vi "Run RT Sequence.vi"(0 "Sequence Context":T1, 1 "RT Sequence File Path":path, 2 "Gateway IP Address":string, 3 "Target (\"\": Auto-assign)":string, 4 "Sequence Timeout (s)":i32=10000, 5 "Step Timeout (ms)":dbl=10000.0, 6 "ParamNames":string[](array[string]), 7 "NumericDataType":string, 8 "ParamValues":string[](array[string]), 10 "ParamTypes":string[](array[string])) -> (14 "Report Text":string, 15 "Numeric Return Value":dbl, 16 "PassFail Return Value":bool, 17 "RT Sequence File Path out":path, 19 "error out":errorcluster)   [LabVIEW 2020, in "ni-veristand-steps-runtime-lib.lvlib"]
uses:
  ni-veristand-steps-runtime-lib.lvlib
  <vilib>/addons/TestStand/_TSLegacy.llb/LabVIEW Test - Sequence Context.ctl
  NationalInstruments.VeriStand.DataTypes
  <vilib>/NI VeriStand/Execution/SequenceExecutionInterface/Sequence Execution State.ctl
  <vilib>/NI VeriStand/Execution/SequenceExecutionInterface/NI_VS Sequence Execution Interface.lvlib
panel:
  out "Session Name out":string
  out "ms time elapsed (debug)":u32
  out "Timed out?":bool
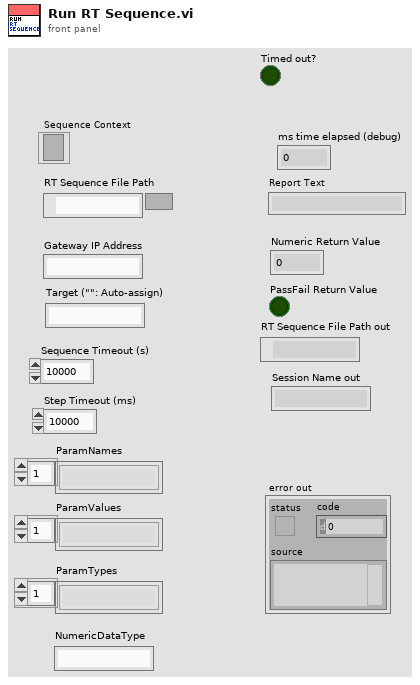
[diagram p1: front panel]
types:
  T1 = typedef "LabVIEW Test - Sequence Context.ctl" = refnum<k7>
  T2 = typedef "NI_VS Sequence Execution Interface.lvlib/Sequence Input Assignment Ref.ctl" = refnum<k24>
  T3 = typedef "NI_VS Sequence Execution Interface.lvlib/Sequence Call Ref.ctl" = refnum<k24>
  T4 = typedef "NI_VS Sequence Execution Interface.lvlib/Stimulus Profile Session Ref.ctl" = refnum<k24>
  T5 = typedef "TestStand - Status Monitor.ctl" = cluster{"Sequence Context":refnum<k7>, "Execution":refnum<k7>, "Termination Monitor":refnum<k7>}
  T6 = typedef "NI_VS Sequence Execution Interface.lvlib/Sequence Execution State.ctl" = enum16{"Idle", "Running", "SingleStepping", "Paused", "Stopped"}
  T7 = typedef "NI_VS Sequence Execution Interface.lvlib/Data Value Ref.ctl" = refnum<k24>
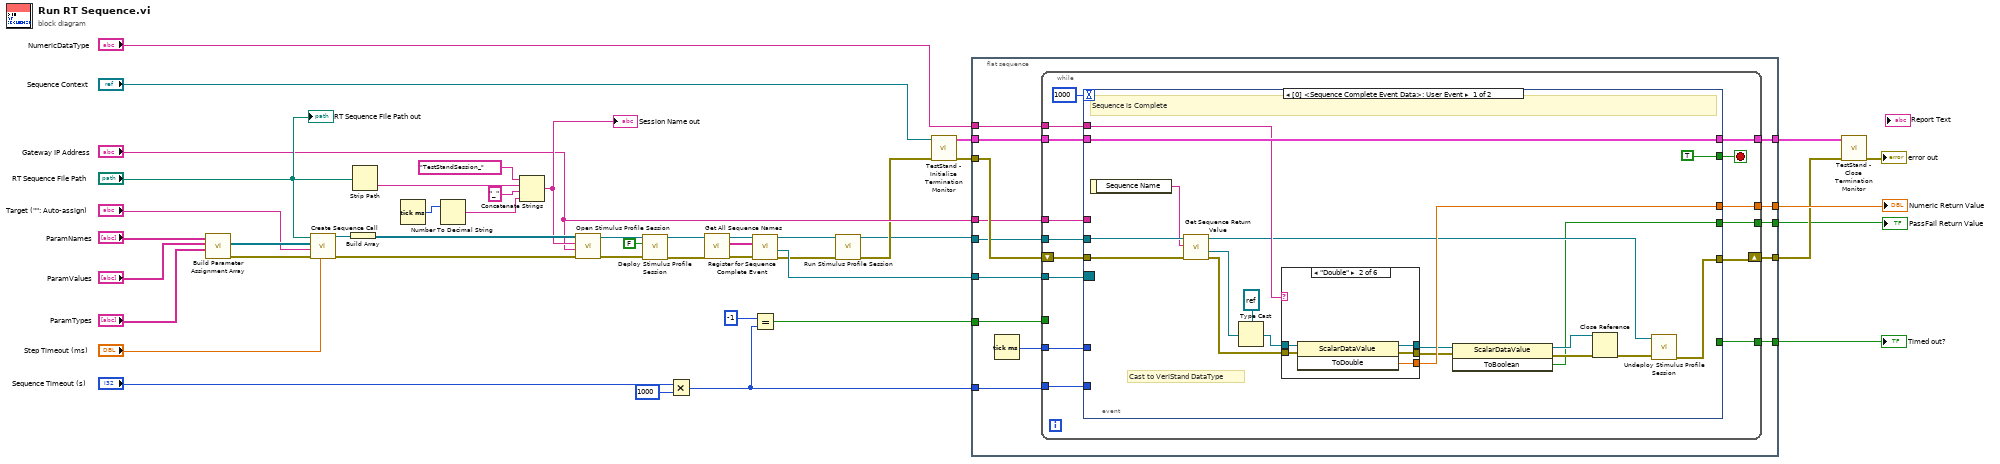
[diagram p0: block diagram]
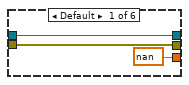
[diagram p2: hidden frame]
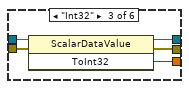
[diagram p3: hidden frame]
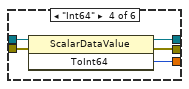
[diagram p4: hidden frame]
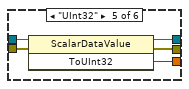
[diagram p5: hidden frame]
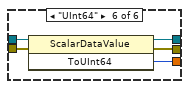
[diagram p6: hidden frame]
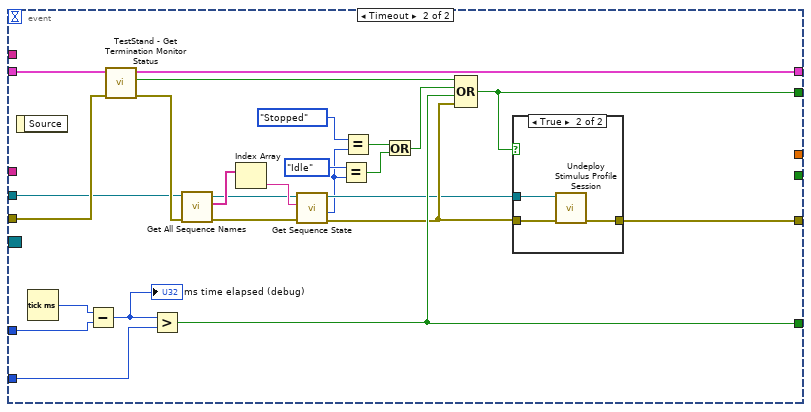
[diagram p7: hidden frame]
diagram:
  n1 = call "Build Parameter Assignment Array.vi"("ParamTypes"="ParamTypes", "ParamValues"="ParamValues", "ParamNames"="ParamNames") -> ("error out"=w43:errorcluster, "Sequence Parameter Assignment refs"=w42:T2[])  [unwired: 7 in]
  n2 = call <vilib>:"Create Sequence Call.vi"("Timeout ms (10000)"="Step Timeout (ms)", "error in (no error)"=w43, "Target (\"\": Auto-assign)"="Target (\"\": Auto-assign)", "Parameter Assignments"=w42, "Sequence File Path"="RT Sequence File Path") -> ("error out"=w11:errorcluster, "Sequence Call Ref"=w40:T3)  [unwired: 5 in]
  n3 = Build Array(w40) -> (w39:T3[])
  n4 = Strip Path(path="RT Sequence File Path") -> (name=w12:string)  [unwired: 1 out]
  n5 = Tick Count (ms)() -> (millisecond timer value=w8:u32)
  n6 = Number To Decimal String(number=w8) -> (decimal integer string=w7:string)  [unwired: 1 in]
  n7 = Concatenate Strings("TestStandSession_" ("Session Name"), w12, "_" ("string"), w7) -> (w14:string)
  "Session Name out" <- w14
  n8 = call <vilib>:"Open Stimulus Profile Session.vi"("error in (no error)"=w11, "Gateway IP Address (\"\": localhost)"="Gateway IP Address", "Session Name"=w14, "Sequence Calls"=w39) -> ("error out"=w36:errorcluster, "Session Ref"=w37:T4)  [unwired: 6 in]
  n9 = call <vilib>:"Deploy Stimulus Profile Session.vi"("error in (no error)"=w36, "Auto-Start (T)"=FALSE, "Session Ref in"=w37) -> ("error out"=w35:errorcluster, "Session Ref out"=w34:T4)  [unwired: 6 in, 1 out]
  n10 = Multiply(x="Sequence Timeout (s)", y=1000) -> (x*y=w26:i32)
  n11 = call <vilib>:"Get All Sequence Names.vi"("error in (no error)"=w35, "Session Ref in"=w34) -> ("error out"=w24:errorcluster, "Sequence Names out"=w22:string[], "Session Ref out"=w23:T4)  [unwired: 7 in]
  n12 = call <vilib>:"Register for Sequence Complete Event.vi"("error in (no error)"=w24, "Sequence Names"=w22, "Session Ref in"=w23) -> ("error out"=w3:errorcluster, "Event Registration Refnum"=w9:refnum<event-registration>, "Session Ref out"=w4:T4)  [unwired: 4 in, 2 out]
  n13 = Equal?(x=-1, y=w26) -> (x = y?=w29:bool)
  n14 = call <vilib>:"Run Stimulus Profile Session.vi"("error in (no error)"=w3, "Session Ref in"=w4) -> ("error out"=w2:errorcluster, "Session Ref out"=w1:T4)  [unwired: 8 in]
  n15 = call <vilib>:"TestStand - Initialize Termination Monitor.vi"("error in (no error)"=w2, "Sequence Context In"="Sequence Context") -> ("error out"=w32:errorcluster, "Status Monitor Out"=w31:T5)  [unwired: 8 in]
  n16 = flat-sequence {
    tunnel: w32 -> [w60]
    tunnel: w31 -> [w59]
    tunnel: w29 -> [w58]
    tunnel: w26 -> [w57]
    tunnel: w1 -> [w56]
    tunnel: w9 -> [w55]
    tunnel: [w54] -> w18
    tunnel: [w53] -> w21
    tunnel: "NumericDataType" -> [w51]
    tunnel: [w50] -> w19
    tunnel: [w49] -> w16
    tunnel: [w48] -> w17
    tunnel: "Gateway IP Address" -> [w47]
    frame #0 {
      n17 = Tick Count (ms)() -> (millisecond timer value=w52:u32)
      n18 = while {
        tunnel: w59 -> [w69]
        tunnel: w57 -> [w66]
        tunnel: w58 -> [_]
        shift-right: [w71] -> w54
        shift-left: w60 -> [w75]
        tunnel: w56 -> [w74]
        tunnel: w55 -> [w73]
        tunnel: [w68] -> w53
        tunnel: w52 -> [w67]
        tunnel: w51 -> [w65]
        tunnel: [w64] -> w50
        tunnel: [w63] -> w49
        tunnel: [w62] -> w48
        tunnel: w47 -> [w61]
        stop <- w72 stop-if-true
        n19 = event shown="[0] <Sequence Complete Event Data>: User Event" {
          selector: w73 -> [_ _]
          dyn-events: _ -> [_ _]
          timeout: 1000 -> [_ _]
          tunnel: w75 -> [w92 w146]
          tunnel: w74 -> [w91 w135]
          tunnel: [TRUE w137] -> w72
          tunnel: [w77 w138] -> w71
          tunnel: w69 -> [w93 w147]
          tunnel: [w93 w145] -> w68
          tunnel: w67 -> [_ w143]
          tunnel: w66 -> [_ w141]
          tunnel: w65 -> [w85 _]
          tunnel: [w84 _] -> w64
          tunnel: [w76 _] -> w63
          tunnel: [_ w139] -> w62
          tunnel: w61 -> [_ _]
          event User Event {
            # "Cast to VeriStand DataType"
            # "Sequence is Complete"
            n20 = event-data() -> ("Sequence Name"=w90:string)  [unwired: 1 in]
            n21 = call <vilib>:"Get Sequence Return Value.vi"("error in (no error)"=w92, "Sequence Name"=w90, "Session Ref in"=w91) -> ("error out"=w87:errorcluster, "Data Value Ref"=w88:T7, "Session Ref out"=w78:T4)  [unwired: 5 in, 1 out]
            n22 = Type Cast(type=refnum<k24> refnum ("Node"), x=w88) -> (*(type *) &x=w86:refnum<k24>)
            n23 = case shown="\"Double\"" w85 {
              tunnel: [w95 w102 w107 w112 w117 w122] -> w83
              tunnel: [w96 w101 w106 w111 w116 w121] -> w82
              tunnel: [nan ("ToDouble") w100 w105 w110 w115 w118] -> w84
              tunnel: w86 -> [w96 w99 w103 w109 w113 w119]
              tunnel: w87 -> [w95 w98 w104 w108 w114 w120]
              frame Default {
              }
              frame "Double" {
                n24 = invoke class="ScalarDataValue" method="ToDouble"(reference=w99, error in=w98) -> (reference out=w101:refnum<k24>, error out=w102:errorcluster, "ToDouble"=w100:dbl)  [unwired: 1 in]
              }
              frame "Int32" {
                n25 = invoke class="ScalarDataValue" method="ToInt32"(reference=w103, error in=w104) -> (reference out=w106:refnum<k24>, error out=w107:errorcluster, "ToInt32"=w105:i32)  [unwired: 1 in]
              }
              frame "Int64" {
                n26 = invoke class="ScalarDataValue" method="ToInt64"(reference=w109, error in=w108) -> (reference out=w111:refnum<k24>, error out=w112:errorcluster, "ToInt64"=w110:i64)  [unwired: 1 in]
              }
              frame "UInt32" {
                n27 = invoke class="ScalarDataValue" method="ToUInt32"(reference=w113, error in=w114) -> (reference out=w116:refnum<k24>, error out=w117:errorcluster, "ToUInt32"=w115:u32)  [unwired: 1 in]
              }
              frame "UInt64" {
                n28 = invoke class="ScalarDataValue" method="ToUInt64"(reference=w119, error in=w120) -> (reference out=w121:refnum<k24>, error out=w122:errorcluster, "ToUInt64"=w118:u64)  [unwired: 1 in]
              }
            }
            n29 = invoke class="ScalarDataValue" method="ToBoolean"(reference=w82, error in=w83) -> (reference out=w80:refnum<k24>, error out=w81:errorcluster, "ToBoolean"=w76:bool)  [unwired: 1 in]
            n30 = Close Reference(reference=w80, error in (no error)=w81) -> (error out=w79:errorcluster)
            n31 = call <vilib>:"Undeploy Stimulus Profile Session.vi"("error in (no error)"=w79, "Session Ref in"=w78) -> ("error out"=w77:errorcluster)  [unwired: 8 in, 1 out]
          }
          event Timeout {
            n32 = event-data() -> ()  [unwired: 1 in, 1 out]
            n33 = Tick Count (ms)() -> (millisecond timer value=w144:u32)
            n34 = Subtract(x=w144, y=w143) -> (x-y=w142:u32)
            "ms time elapsed (debug)" <- w142
            n35 = call <vilib>:"TestStand - Get Termination Monitor Status.vi"("error in (no error)"=w146, "Status Monitor In"=w147) -> ("error out"=w136:errorcluster, "Terminating or Aborting"=w140:bool, "Status Monitor Out"=w145:T5)  [unwired: 7 in]
            n36 = Greater?(x=w142, y=w141) -> (0:w139:bool)
            n37 = call <vilib>:"Get All Sequence Names.vi"("error in (no error)"=w136, "Session Ref in"=w135) -> ("error out"=w134:errorcluster, "Sequence Names out"=w133:string[], "Session Ref out"=w131:T4)  [unwired: 7 in]
            n38 = Index Array(array=w133) -> (element=w132:string)  [unwired: 1 in]
            n39 = call <vilib>:"Get Sequence State.vi"("error in (no error)"=w134, "Sequence Name"=w132, "Session Ref in"=w131) -> ("error out"=w130:errorcluster, "State"=w127:T6, "Session Ref out"=w129:T4)  [unwired: 5 in, 1 out]
            n40 = Equal?(x=Sequence_Execution_State."Idle", y=w127) -> (x = y?=w124:bool)
            n41 = Equal?(x=Sequence_Execution_State."Stopped", y=w127) -> (x = y?=w125:bool)
            n42 = Or(x=w125, y=w124) -> (x .or. y?=w123:bool)
            n43 = Compound Arithmetic op=OR(w140, w123, w139, w130) -> (w137:bool)
            n44 = case shown="True" w137 {
              tunnel: [w148 w151] -> w138
              tunnel: w130 -> [w148 w150]
              tunnel: w129 -> [_ w149]
              frame False {
              }
              frame True {
                n45 = call <vilib>:"Undeploy Stimulus Profile Session.vi"("error in (no error)"=w150, "Session Ref in"=w149) -> ("error out"=w151:errorcluster)  [unwired: 8 in, 1 out]
              }
            }
          }
        }
      }
    }
  }
  n46 = call <vilib>:"TestStand - Close Termination Monitor.vi"("error in (no error)"=w18, "Status Monitor In"=w21) -> ("error out"=→"error out":errorcluster)  [unwired: 9 in]
  "Timed out?" <- w17
  "Numeric Return Value" <- w19
  "PassFail Return Value" <- w16
  "RT Sequence File Path out" <- "RT Sequence File Path"
